vi "MBT_CreateLogFileDir.vi"(11 "path":path) -> (3 "appended path":path)   [LabVIEW 2012, in "MBT_ModbusTester.lvlib"]
uses:
  MBT_ModbusTester.lvlib
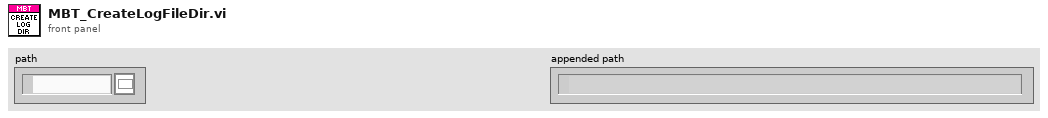
[diagram p1: front panel]
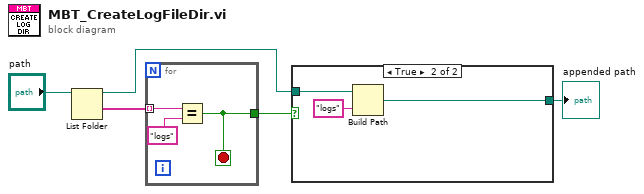
[diagram p0: block diagram]
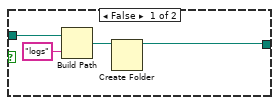
[diagram p2: hidden frame]
diagram:
  n1 = List Folder(path="path") -> (path out=w1:path, folder names=w4:string[])  [unwired: 3 in, 2 out]
  n2 = for {
    tunnel: w4 -> [w8] mode=indexing
    tunnel: [w6] -> w5
    stop <- w6 stop-if-true
    n3 = Equal?(x=w8, y="logs") -> (x = y?=w6:bool)
  }
  n4 = case shown="True" w5 {
    tunnel: [w10 w14] -> w3
    tunnel: w1 -> [w9 w13]
    frame False {
      n5 = Build Path(base path=w9, name or relative path="logs") -> (appended path=w11:path)
      n6 = Create Folder(path (use dialog)=w11) -> (created path=w10:path)  [unwired: 2 in, 2 out]
    }
    frame True {
      n7 = Build Path(base path=w13, name or relative path="logs") -> (appended path=w14:path)
    }
  }
  "appended path" <- w3
